vi "Restore sequence from stacked tiff.vi"(6 "Milliseconds per frame":dbl format="%.2f", 7 "error in":errorcluster, 9 "Sequence files handle":T1, 10 "Directory path":path) -> (0 "error out":errorcluster, 3 "Last frame number written out":u32)   [LabVIEW 2011]
doc: "Takes a sequence of individual image files (e.g., TIFFs) or a SEQ file and loads it in to an acquisition file.\n\nINPUTS:\nDirectory name (sequence name with path). If left empty, the program will prompt for name.\nSequence of images.\nFile format (AIPD as default)"
uses:
  Sequence files handle.ctt
  Seq file v 1/Offset table.ctl
  Seq file v 1/Offset.ctl
  Seq file v 1/file number.ctl
  Header2 file data.ctl
panel:
  out "Image Type":u32(ring) items=["8 bits", "16 bits", "Float", "Complex", "RGB", "HSL"]
  in  "Quit":bool
  out "Frame number":i32(slide) scale=1.0..10.0
  out "File":path
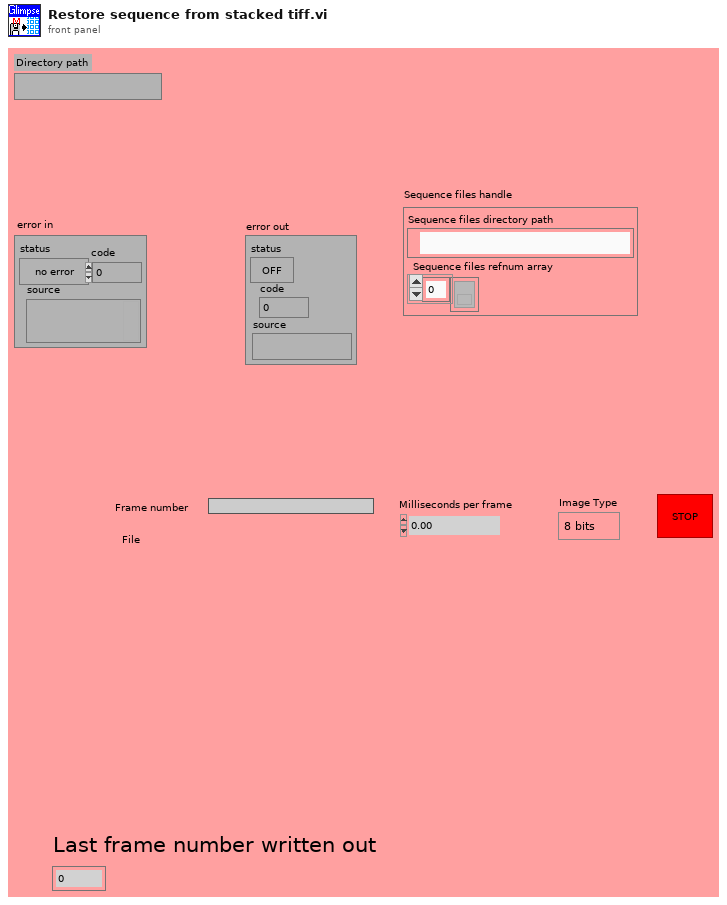
[diagram p1: front panel]
types:
  T1 = typedef "Sequence files handle.ctt" = cluster{"Sequence files directory path":path, "Sequence files refnum array":refnum<file>[]}
  T2 = enum32{"existing file", "new file", "new or existing file", "existing dir", "new dir", "new or existing dir", "existing file (use LLBs)", "new file (use LLBs)", "new or existing file (use LLBs)", "new or existing file or directory (use LLBs)"}
  T3 = typedef "Offset table.ctl" = cluster{"offset":T4, "file number":T5}[]
  T4 = typedef "Offset.ctl" = i32
  T5 = typedef "file number.ctl" = u8
  T6 = typedef "IMAQ Image.ctl" = refnum<image>
  T7 = typedef "Header2 file data.ctl" = cluster{"Camera":string, "Microscope":string, "Microscope software version":string, "Laser names":string[], "Filter names":string[], "Lasers array":u16[][], "Filter array":u16[], "Flow rate array":dbl[], "Temperature array":dbl[], "Field array":u16[], "Is header2 info present?":bool, "Description Info":string, "Stage xyz array":dbl[][]}
  T8 = typedef "Header file data.ctl" = cluster{"Frames Acquired":u32, "Region width":i32, "Region height":i32, "Element 0 of TTB":u32, "time of 1st frame, \nsec since 1/1/04":dbl, "TTB Array (ms)":u32[], "Offsets Array":T3, "Pixel depth":u32}
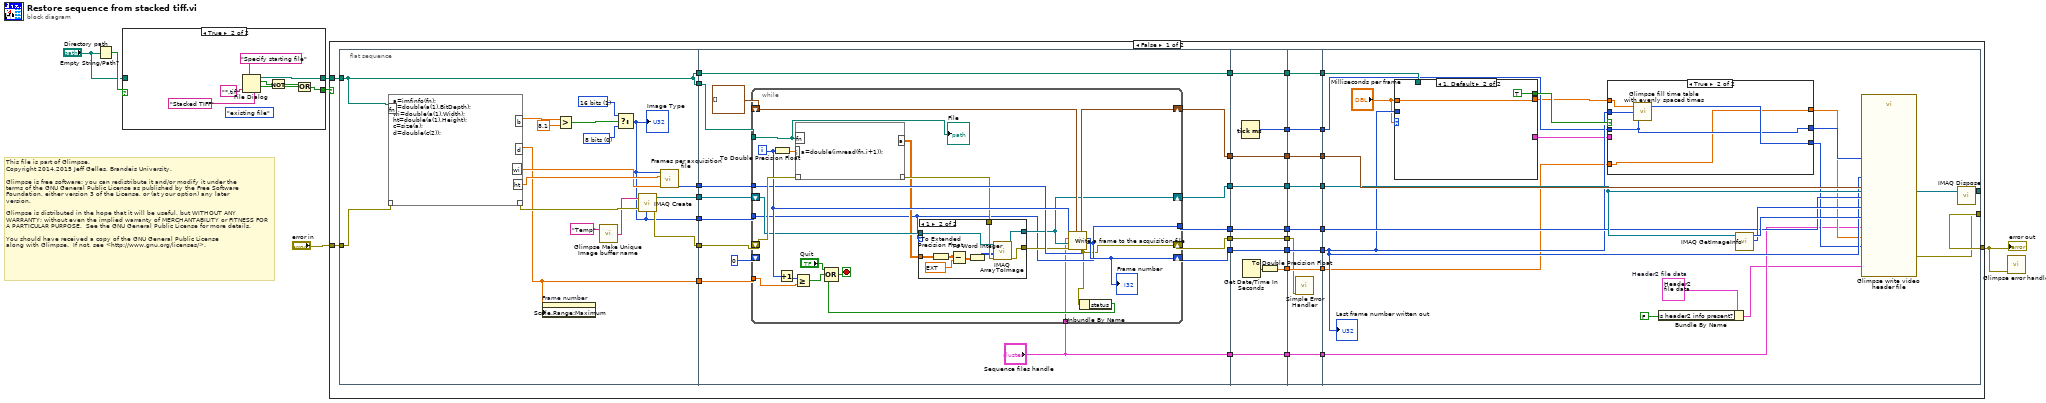
[diagram p0: block diagram]
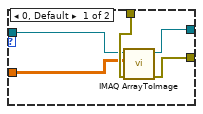
[diagram p2: hidden frame]
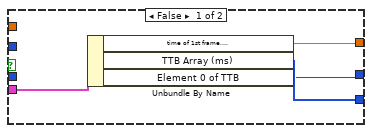
[diagram p3: hidden frame]
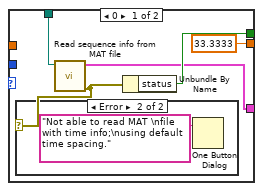
[diagram p4: hidden frame]
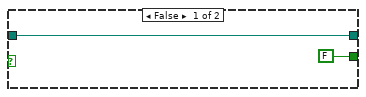
[diagram p7: hidden frame]
diagram:
  # "This file is part of Glimpse. \nCopyright 2014,2015 Jeff Gelles, Brandeis University.    \n\nGlimpse is free software: you can redistribute it and/or modify it under the \nterms of the GNU General Public License as published by the Free Software \nFoundation, either version 3 of the License, or (at your option) any later \nversion.\n\nGlimpse is distributed in the hope that it will be useful, but WITHOUT ANY \nWARRANTY; without even the implied warranty of MERCHANTABILITY or FITNESS FOR \nA PARTICULAR PURPOSE.  See the GNU General Public License for more details.\n\nYou should have received a copy of the GNU General Public License\nalong with Glimpse.  If not, see <http://www.gnu.org/licenses/>."
  n1 = Empty String/Path?(string/path="Directory path") -> (empty?=w6:bool)
  n2 = case shown="True" w6 {
    tunnel: [w8 w16] -> w4
    tunnel: "Directory path" -> [w8 _]
    tunnel: [FALSE ("cancelled") w11] -> w3
    frame False {
    }
    frame True {
      (unwired) T2."existing file" ("select mode (2)")
      n3 = File Dialog(4:"Stacked TIFF" ("pattern label"), 6:"*.tif" ("pattern"), 7:"Specify starting file" ("prompt")) -> (1:w12:bool, 2:w14:bool, 3:w16:path)  [unwired: 1 in, 4 out]
      n4 = Not(x=w14) -> (.not. x?=w13:bool)
      n5 = Or(x=w13, y=w12) -> (x .or. y?=w11:bool)
    }
  }
  n6 = case shown="False" w3 {
    tunnel: w4 -> [w51 _]
    tunnel: "error in" -> [w50 w177]
    tunnel: [w49 w177] -> w1
    frame False {
      n7 = flat-sequence {
        tunnel: w51 -> [w54]
        tunnel: w50 -> [w68]
        tunnel: [w64] -> w48
        tunnel: [w56] -> w42
        tunnel: [w54] -> w41
        tunnel: [w53] -> w40
        tunnel: [w55] -> w39
        tunnel: [w52] -> w38
        tunnel: [w54] -> w35
        tunnel: w48 -> [w83]
        tunnel: [w81] -> w47
        tunnel: [w78] -> w46
        tunnel: [w80] -> w45
        tunnel: [w77] -> w44
        tunnel: w42 -> [w76]
        tunnel: w41 -> [w75]
        tunnel: w40 -> [w74]
        tunnel: w39 -> [w73]
        tunnel: w38 -> [w72]
        tunnel: [w71] -> w37
        tunnel: [w70] -> w36
        tunnel: w35 -> [w70]
        tunnel: ["Sequence files handle"] -> w19
        tunnel: w47 -> [w129]
        tunnel: [w129] -> w34
        tunnel: w46 -> [w128]
        tunnel: [w128] -> w32
        tunnel: w45 -> [w125]
        tunnel: [w125] -> w30
        tunnel: w44 -> [w127]
        tunnel: [w127] -> w29
        tunnel: [w124] -> w27
        tunnel: [w123] -> w25
        tunnel: w37 -> [w122]
        tunnel: [w122] -> w23
        tunnel: [w121] -> w21
        tunnel: w36 -> [w121]
        tunnel: w19 -> [w120]
        tunnel: [w120] -> w18
        tunnel: w34 -> [w138]
        tunnel: [w138] -> w33
        tunnel: w32 -> [w137]
        tunnel: [w137] -> w31
        tunnel: w30 -> [w131]
        tunnel: w29 -> [w136]
        tunnel: [w136] -> w28
        tunnel: w27 -> [w135]
        tunnel: [w135] -> w26
        tunnel: w25 -> [w132]
        tunnel: [w132] -> w24
        tunnel: w23 -> [w134]
        tunnel: [w134] -> w22
        tunnel: w21 -> [w133]
        tunnel: [w133] -> w20
        tunnel: w18 -> [w130]
        tunnel: [w130] -> w17
        tunnel: [w159] -> w49
        tunnel: w33 -> [w151]
        tunnel: w31 -> [w158]
        tunnel: w28 -> [w155]
        tunnel: w26 -> [w150]
        tunnel: w24 -> [w146]
        tunnel: [w155] -> w43
        tunnel: w22 -> [w154]
        tunnel: w20 -> [w153]
        tunnel: w17 -> [w142]
        frame #0 {
          w60 = u32 1 items=["8 bits", "16 bits", "Float", "Complex", "RGB", "HSL"] ("Image Type")
          w59 = u32 0 items=["8 bits", "16 bits", "Float", "Complex", "RGB", "HSL"] ("Image Type")
          n8 = script code="a=imfinfo(fn);\nb=double(a(1).BitDepth);\nwi=double(a(1).Width);\nht=double(a(1).Height);\nc=size(a);\nd=double(c(2));"("??"=w68, "fn"=w54) -> ("??"=w65:errorcluster, "b"=w63:dbl, "d"=w53:dbl, "wi"=w66:dbl, "ht"=w67:dbl)
          n9 = property on="Frame number" class="Slide (strict)"("Scale.Range:Maximum"=w53) -> ()  [unwired: 2 in, 2 out]
          n10 = Greater?(x=w63, y=8.1) -> (0:w61:bool)
          n11 = call "Glimpse Make Unique Image buffer name.vi"("Buffer  base name"="Temp") -> ("Image Name"=w58:string)  [unwired: 1 out]
          n12 = Select(t=w60, s=w61, f=w59) -> (s? t:f=w52:u32)
          "Image Type" <- w52
          n13 = call "IMAQ Create"("Image Name"=w58, "Image Type"=w52, "error in (no error)"=w65) -> ("New Image"=w56:T6, "error out"=w64:errorcluster)  [unwired: 1 in, 1 out]
          n14 = call "Frames per axquisition file.vi"("Output frame width"=w66, "Output frame height"=w67, "Pixel depth"=w52) -> ("Frames per acquisition file"=w55:i32)  [unwired: 3 in, 1 out]
        }
        frame #1 {
          n15 = while {
            shift-left: 0 -> [_]
            shift-right: [w105] -> w81
            shift-left: w83 -> [w102]
            shift-right: [w86] -> w80
            shift-right: [w103] -> w78
            shift-left: T3 [] ("Offset table out") -> [w104]
            shift-right: [w93] -> w77
            shift-left: w76 -> [w92]
            tunnel: w75 -> [w100]
            tunnel: w74 -> [w87]
            tunnel: w73 -> [w95]
            tunnel: w72 -> [w89]
            tunnel: [w89] -> w71
            tunnel: "Sequence files handle" -> [w84]
            i -> [w99]
            stop <- w96 stop-if-true
            n16 = To Double Precision Float(number=w99) -> (double precision float=w101:dbl)
            n17 = Increment(x=w99) -> (x+1=w88:i32)
            n18 = Greater Or Equal?(x=w88, y=w87) -> (x >= y?=w97:bool)
            n19 = script code="a=double(imread(fn,i+1));"("??"=w102, "fn"=w100, "i"=w101) -> ("??"=w91:errorcluster, "a"=w90:dbl[][])
            n20 = case shown="1" w89 {
              tunnel: [w109 w119] -> w94
              tunnel: [w110 w118] -> w93
              tunnel: w92 -> [w106 w117]
              tunnel: w91 -> [w108 w116]
              tunnel: w90 -> [w107 w115]
              frame 0, Default {
                n21 = call "IMAQ ArrayToImage"("error in (no error)"=w108, "Image Pixels (U8)"=w107, "Image"=w106) -> ("error out"=w109:errorcluster, "Image Out"=w110:T6)  [unwired: 3 in, 4 out]
              }
              frame 1 {
                n22 = To Extended Precision Float(1:w115) -> (0:w114:ext[][])
                n23 = Subtract(x=w114, y=ext 32768.0) -> (x-y=w113:ext[][])
                n24 = To Word Integer(number=w113) -> (16bit integer=w111:i16[][])
                n25 = call "IMAQ ArrayToImage"("error in (no error)"=w116, "Image Pixels (I16)"=w111, "Image"=w117) -> ("error out"=w119:errorcluster, "Image Out"=w118:T6)  [unwired: 3 in, 4 out]
              }
            }
            n26 = call "Write a frame to the acquisition file.vi"("Pixel depth"=w89, "Frames per acquisition file"=w95, "Offset table in"=w104, "error in"=w94, "Image In"=w93, "Sequence files handle"=w84, "Last frame number written in"=w99) -> ("error out"=w86:errorcluster, "Last frame number written out"=w105:u32, "Offset table out"=w103:T3)  [unwired: 2 out]
            "Frame number" <- w105
            n27 = Unbundle By Name(w86) -> ("status"=w85:bool)
            n28 = Compound Arithmetic op=OR("Quit", w97, w85) -> (w96:bool)
            "File" <- w100
          }
        }
        frame #2 {
          n29 = Tick Count (ms)() -> (millisecond timer value=w124:u32)
          n30 = Get Date/Time In Seconds() -> (seconds since 1Jan1904=w126:timestamp)
          n31 = To Double Precision Float(number=w126) -> (double precision float=w123:dbl)
        }
        frame #3 {
          n32 = call <vilib>:"Simple Error Handler.vi"("error in (no error)"=w131) -> ()  [unwired: 1 in, 8 out]
        }
        frame #4 {
          w141 = T7 {"Camera"="", "Microscope"="", "Microscope software version"="", "Laser names"=[], "Filter names"=[], "Lasers array"=[], "Filter array"=[], "Flow rate array"=[], "Temperature array"=[], "Field array"=[], "Is header2 info present?"=FALSE, "Description Info"="", "Stage xyz array"=[]}  # Header2 file data
          n33 = case shown="1, Default" "Milliseconds per frame" {
            tunnel: w151 -> [_ _]
            tunnel: w153 -> [w173 _]
            tunnel: [w171 TRUE ("status")] -> w152
            tunnel: [w170 _] -> w145
            tunnel: [33.3333 ("Milliseconds per frame") w175] -> w144
            tunnel: "Milliseconds per frame" -> [_ w175]
            frame 0 {
              n34 = call "Read sequence info from MAT file.vi"("Movie file name"=w173) -> ("error out"=w172:errorcluster, "Header file data"=w170:T8)  [unwired: 1 in, 8 out]
              n35 = case shown="Error" w172 {
                frame No Error {
                }
                frame Error {
                  n36 = One Button Dialog(message="Not able to read MAT \nfile with time info;\nusing default time spacing.") -> ()  [unwired: 2 out]
                }
              }
              n37 = Unbundle By Name(w172) -> ("status"=w171:bool)
            }
            frame 1, Default {
            }
          }
          n38 = case shown="True" w152 {
            tunnel: [w161 w168] -> w149
            tunnel: w144 -> [_ w167]
            tunnel: w151 -> [_ w166]
            tunnel: w150 -> [_ w165]
            tunnel: [w162 w164] -> w147
            tunnel: [w160 w165] -> w148
            tunnel: w146 -> [_ w164]
            tunnel: w145 -> [w163 _]
            frame False {
              n39 = Unbundle By Name(w163) -> ("time of 1st frame, \nsec since 1/1/04"=w162:dbl, "TTB Array (ms)"=w161:u32[], "Element 0 of TTB"=w160:u32)
            }
            frame True {
              n40 = call "Glimpse fill time table with evenly spaced times.vi"("Element 0 of TTB"=w165, "Number of frames in sequence"=w166, "Milliseconds per frame"=w167) -> ("TTB Array"=w168:u32[])  [unwired: 2 out]
            }
          }
          n41 = Bundle By Name(cluster=w141, "Is header2 info present?"=FALSE) -> (w140:T7)
          n42 = call "IMAQ GetImageInfo"("Image"=w155) -> ("Y Resolution"=w156:i32, "X Resolution"=w157:i32)  [unwired: 1 in, 8 out]
          n43 = call "Glimpse write video header file.vi"("Number of frames"=w151, "Sequence files handle"=w142, "Pixel depth\n(0=8 bit; 1= 16 bit)"=w154, "TTB Array"=w149, "Offsets Array"=w158, "Header2 file data"=w140, "Region width"=w157, "Region height"=w156, "Element 0 of TTB"=w148, "time of 1st frame, \nsec since 1/1/04"=w147) -> ("error out"=w159:errorcluster)  [unwired: 9 in]
          "Last frame number written out" <- w151
        }
      }
      n44 = call "IMAQ Dispose"("Image"=w43) -> ()  [unwired: 2 in, 4 out]
    }
    frame True {
    }
  }
  "error out" <- w1
  n45 = call "Glimpse error handler.vi"("error in"=w1) -> ()  [unwired: 1 in, 6 out]
